vi "N5765A_ReadCurrentStandalone.vi"(8 "error in (no error)":errorcluster, 11 "VISA resource name":refnum<visa-resource-name>="PS2") -> (0 "error out":errorcluster, 2 "Measurement":dbl=-0.0009589195 format="%^.3e")   [LabVIEW 2015]
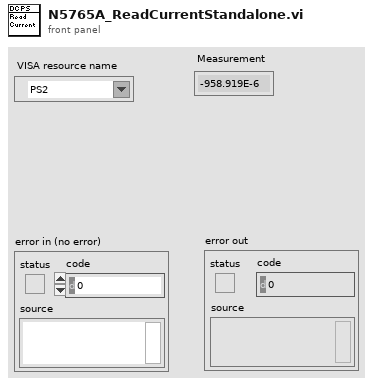
[diagram p1: front panel]
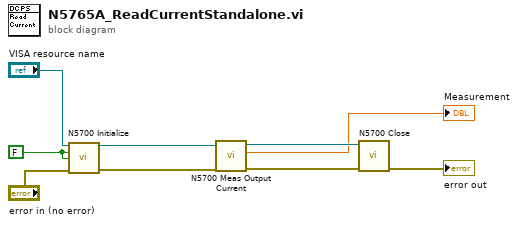
[diagram p0: block diagram]
diagram:
  w8 = FALSE ("ID Query? (T: Yes)")
  n1 = call <instrlib>:"N5700 Initialize.vi"("VISA name"="VISA resource name", "ID Query (T)"=w8, "Reset (T)"=w8, "error in (no error)"="error in (no error)") -> ("VISA out"=w5:refnum<visa-resource-name>, "error out"=w6:errorcluster)  [unwired: 10 in]
  n2 = call <instrlib>:"N5700 Meas Output Current.vi"("error"=w6, "VISA"=w5) -> ("error out"=w4:errorcluster, "Output Current"=→"Measurement":dbl, "VISA out"=w3:refnum<visa-resource-name>)  [unwired: 4 in]
  n3 = call <instrlib>:"N5700 Close.vi"("error"=w4, "VISA name"=w3) -> ("error out"=→"error out":errorcluster)  [unwired: 6 in]
